vi "Write avail logged tags table.vi"(8 "error in (no error)":errorcluster, 10 "avail logged tags table":refnum<vi>, 11 "TDMS datalogger editor node in":refnum<class "TDMS datalogger editor node.lvclass">) -> (0 "error out":errorcluster, 3 "TDMS datalogger editor node out":refnum<class "TDMS datalogger editor node.lvclass">)   [LabVIEW 2015, in "TDMS datalogger editor node.lvclass"]
uses:
  TDMS datalogger editor node.lvclass
  TDMS datalogger editor node.lvclass/TDMS datalogger editor node.ctl
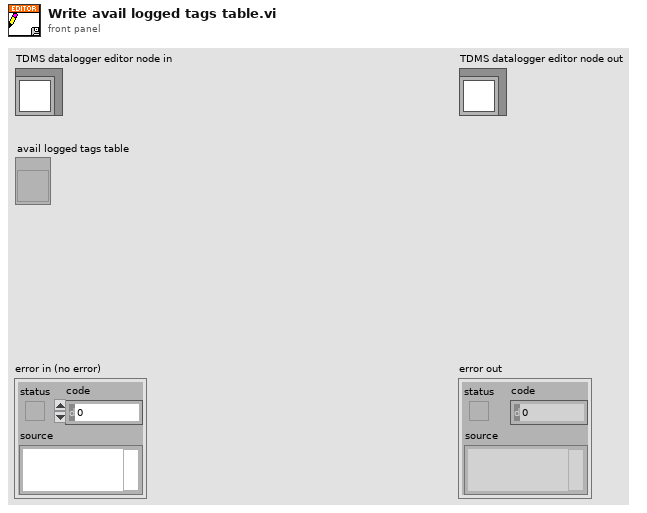
[diagram p1: front panel]
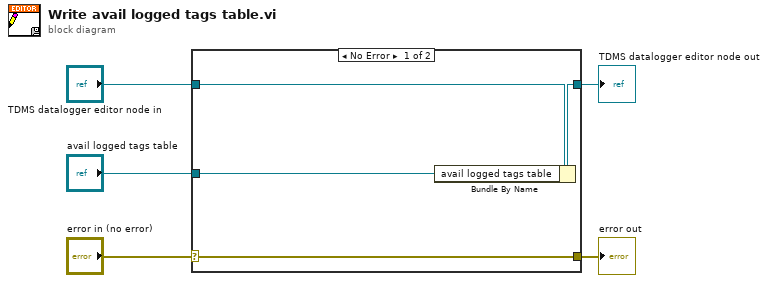
[diagram p0: block diagram]
diagram:
  n1 = case shown="No Error" "error in (no error)" {
    selector: "error in (no error)" -> [w9 w10]
    tunnel: [w9 w10] -> w4
    tunnel: [w7 w11] -> w2
    tunnel: "TDMS datalogger editor node in" -> [w8 w11]
    tunnel: "avail logged tags table" -> [w6 _]
    frame No Error {
      n2 = Bundle By Name(cluster=w8, "avail logged tags table"=w6) -> (w7:refnum<class "TDMS datalogger editor node.lvclass">)
    }
    frame Error {
    }
  }
  "error out" <- w4
  "TDMS datalogger editor node out" <- w2
